vi "ArmPositionToZeroLengthPlanResponse.vi"(1 "Position":T4) -> (0 "ArmPlanResponse":T1 {"WristTrajectory"."Time (ms)" items=["TrajectoryDuration_0ms"=0, "TrajectoryDuration_5ms"=5, "TrajectoryDuration_10ms"=10, "TrajectoryDuration_20ms"=20, "TrajectoryDuration_30ms"=30, "TrajectoryDuration_40ms"=40, "TrajectoryDuration_50ms"=50, "TrajectoryDuration_100ms"=100]; "ExtendTrajectory"."Time (ms)" items=["TrajectoryDuration_0ms"=0, "TrajectoryDuration_5ms"=5, "TrajectoryDuration_10ms"=10, "TrajectoryDuration_20ms"=20, "TrajectoryDuration_30ms"=30, "TrajectoryDuration_40ms"=40, "TrajectoryDuration_50ms"=50, "TrajectoryDuration_100ms"=100]; "ShoulderTrajectory"."Time (ms)" items=["TrajectoryDuration_0ms"=0, "TrajectoryDuration_5ms"=5, "TrajectoryDuration_10ms"=10, "TrajectoryDuration_20ms"=20, "TrajectoryDuration_30ms"=30, "TrajectoryDuration_40ms"=40, "TrajectoryDuration_50ms"=50, "TrajectoryDuration_100ms"=100]})   [LabVIEW 2018]
uses:
  TypeDefs/ArmAbsolutePosition.ctl
  TypeDefs/ArmPlanResponse.ctl
  ArgosLib/MotionProfiling/TypeDefs/TrajectoryPoint.ctl
  <vilib>/Rock Robotics/WPI/ThirdParty/Phoenix-LabVIEW/Motor Controller/Controls/CTRE_Phoenix_MotorControl_TrajectoryPointTimeDur.ctl
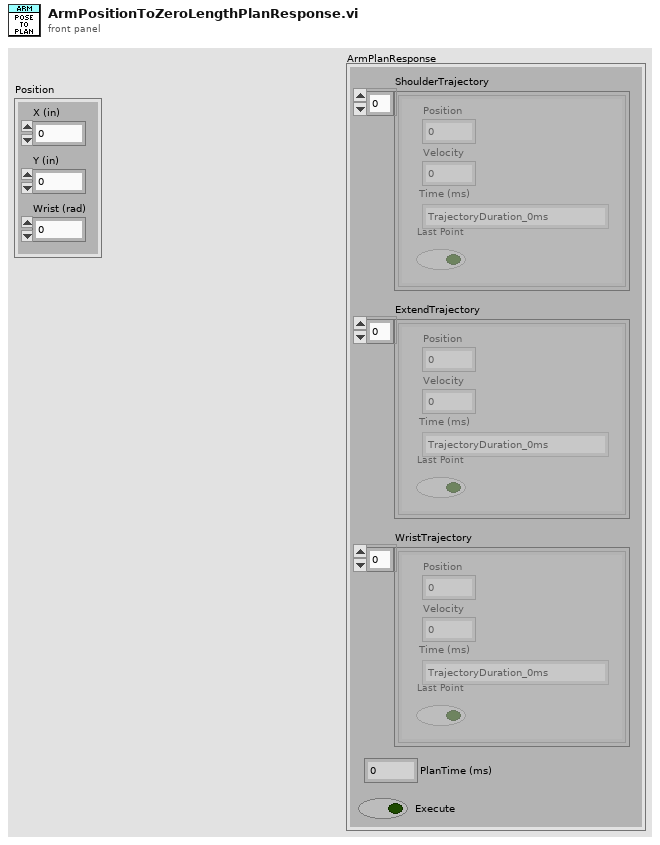
[diagram p1: front panel]
types:
  T1 = typedef "ArmPlanResponse.ctl" = cluster{"ShoulderTrajectory":T2[], "ExtendTrajectory":T2[], "PlanTime (ms)":u32, "Execute":bool, "WristTrajectory":T2[]}
  T2 = typedef "TrajectoryPoint.ctl" = cluster{"Position ":dbl, "Velocity ":dbl, "Time (ms)":T3, "Last Point":bool}
  T3 = typedef "CTRE_Phoenix_MotorControl_TrajectoryPointTimeDur.ctl" = i32
  T4 = typedef "ArmAbsolutePosition.ctl" = cluster{"X (in)":dbl, "Y (in)":dbl, "Wrist (rad)":dbl}
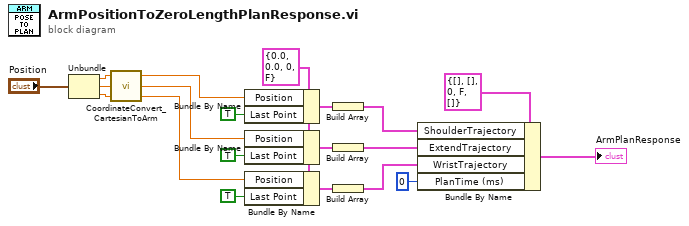
[diagram p0: block diagram]
diagram:
  w9 = T2 {"Position "=0.0, "Velocity "=0.0, "Time (ms)"=0, "Last Point"=FALSE} ("trajectory point")
  n1 = Unbundle("Position") -> ("X (in)"=w20:dbl, "Y (in)"=w19:dbl, "Wrist (rad)"=w18:dbl)
  n2 = call "CoordinateConvert_CartesianToArm.vi"("Wrist (rad)"=w18, "Y (in)"=w19, "X (in)"=w20) -> ("Wrist Angle (rad)"=w7:dbl, "Radius (in)"=w8:dbl, "Shoulder Angle (rad)"=w16:dbl)
  n3 = Bundle By Name(cluster=w9, "Position"=w16, "Last Point"=TRUE) -> (w13:T2)
  n4 = Bundle By Name(cluster=w9, "Position"=w8, "Last Point"=TRUE) -> (w10:T2)
  n5 = Bundle By Name(cluster=w9, "Position"=w7, "Last Point"=TRUE) -> (w12:T2)
  n6 = Build Array(w13) -> (w6:T2[])
  n7 = Build Array(w10) -> (w5:T2[])
  n8 = Build Array(w12) -> (w4:T2[])
  n9 = Bundle By Name(cluster=T1 {"ShoulderTrajectory"=[], "ExtendTrajectory"=[], "PlanTime (ms)"=0, "Execute"=FALSE, "WristTrajectory"=[]} ("ArmPlanResponse"), "ShoulderTrajectory"=w6, "ExtendTrajectory"=w5, "WristTrajectory"=w4, "PlanTime (ms)"=u32 0) -> (→"ArmPlanResponse":T1)
